vi "FPGA_XYMoving.vi"() -> ()   [LabVIEW 2014]
uses:
  <vilib>/rvi/Emulation/niFpgaSctlEmulationGetInTimedLoop.vi
  <vilib>/rvi/Emulation/niFpgaProcessEmulError.vi
  <vilib>/rvi/Memory/Memory_Emulation/nirvimemoryFastEmulation.vi
  <vilib>/rvi/Memory/Memory_Emulation/nirvimemoryEmulation.vi
  <vilib>/rvi/Emulation/niFpgaEmulationIsFPGAContextNoSignature.vi
  <vilib>/rvi/DataTransferAndStorage/Container/Common/niFpgaContainerGetUniqueNameForEmu.vi
  <vilib>/rvi/errors/nirviReportUnexpectedCaseInternalError (U32).vi
  <vilib>/rvi/eio/common/nirviEmuTemplateMethod_errors.vi
  <vilib>/rvi/Emulation/niFpgaGetClockAttributes.vi
  <vilib>/rvi/Emulation/niFpgaEmulationReportErrorSimple.vi
  <vilib>/rvi/occurrence/nirviWaitOnOccurrenceBase.vi
  <vilib>/rvi/Emulation/niFpgaCriticalErrorInLSC.vi
  <vilib>/rvi/DataTransferAndStorage/Container/XNode/niFpgaContainer.xnode
  <vilib>/eio/EIONode/EIONode.xnode
panel:
  out "DIO 0":bool
  out "XPresNum":i32
  out "YPresNum":i32
  in  "YOffset":i16
  in  "XOffset":i16
  in  "YStepIndex":i16
  in  "XStepIndex":i16
  in  "stop":bool
  in  "YNum":i16
  in  "XNum":i16
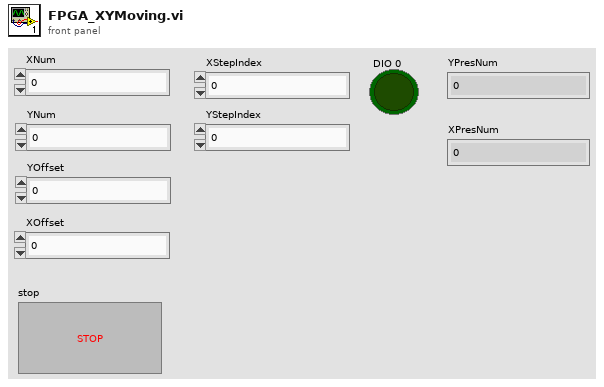
[diagram p1: front panel]
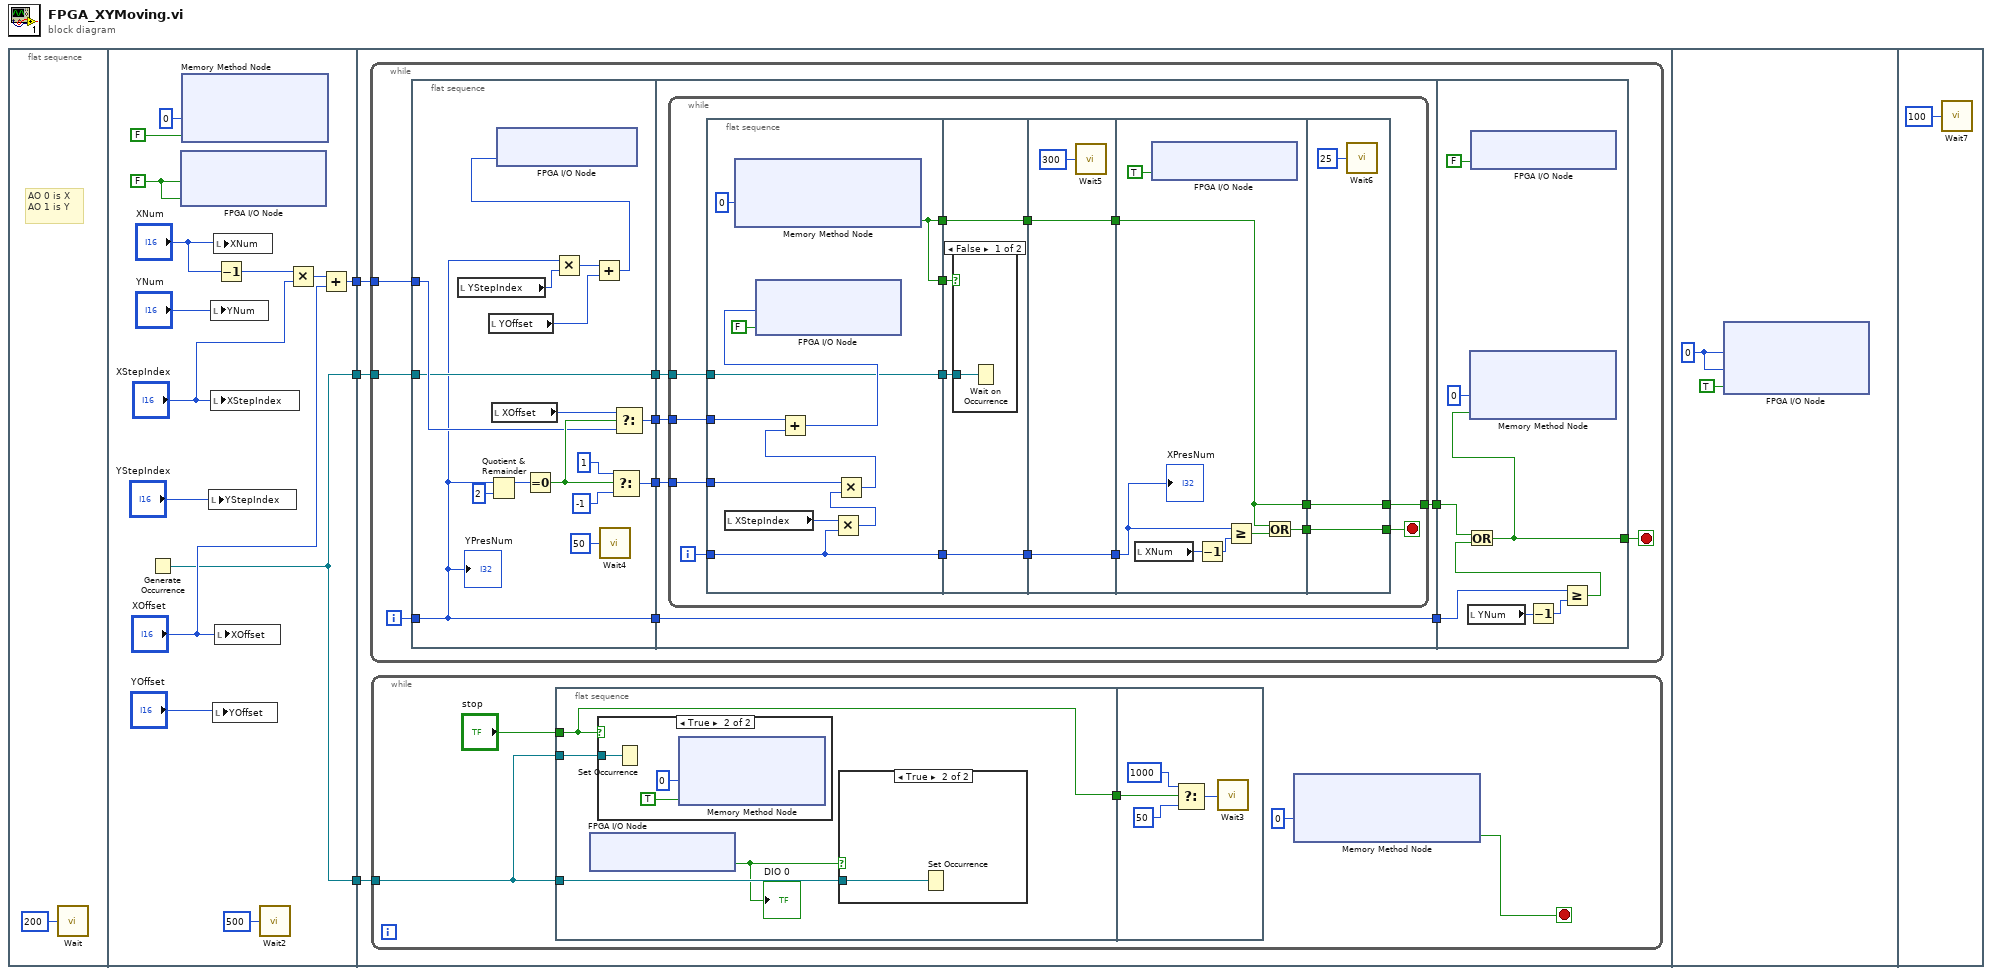
[diagram p0: block diagram]
diagram:
  n1 = flat-sequence {
    tunnel: [w6] -> w3
    tunnel: [w7] -> w2
    tunnel: [w6] -> w1
    tunnel: w3 -> [w21]
    tunnel: w2 -> [w20]
    tunnel: w1 -> [w19]
    frame #0 {
      # "AO 0 is X\nAO 1 is Y"
      n2 = call "Wait"("Count(mSec)"=u32 200) -> ()  [unwired: 1 out]
    }
    frame #1 {
      w5 = FALSE ("Connector0/DIO1")
      n3 = Generate Occurrence() -> (w6:refnum<k4>)
      n4 = xnode "FPGA I/O Node"("Connector0/DIO1"=w5, "Connector0/DIO2"=w5) -> ()  [unwired: 2 in, 2 out]
      n5 = xnode ("Memory Method Node")("Address"=u32 0, "Data"=FALSE) -> ()  [unwired: 1 in, 1 out]
      n6 = local write "YStepIndex"("YStepIndex") -> ()
      n7 = local write "YNum"("YNum") -> ()
      n8 = local write "XStepIndex"("XStepIndex") -> ()
      n9 = local write "YOffset"("YOffset") -> ()
      n10 = local write "XNum"("XNum") -> ()
      n11 = local write "XOffset"("XOffset") -> ()
      n12 = Decrement(x="XNum") -> (x-1=w10:i16)
      n13 = call "Wait2"("Count(uSec)"=u32 500) -> ()  [unwired: 1 out]
      n14 = Multiply(x=w10, y="XStepIndex") -> (x*y=w9:i16)
      n15 = Add(x=w9, y="XOffset") -> (x+y=w7:i16)
    }
    frame #2 {
      n16 = while {
        tunnel: w20 -> [w47]
        tunnel: w19 -> [w44]
        i -> [w48]
        stop <- w39 stop-if-true
        n17 = flat-sequence {
          tunnel: w48 -> [w49]
          tunnel: w47 -> [w60]
          tunnel: [w54] -> w46
          tunnel: [w51] -> w45
          tunnel: w44 -> [w50]
          tunnel: [w50] -> w43
          tunnel: [w49] -> w42
          tunnel: w46 -> [w69]
          tunnel: w45 -> [w68]
          tunnel: w43 -> [w67]
          tunnel: w42 -> [w66]
          tunnel: [w66] -> w41
          tunnel: [w65] -> w40
          tunnel: w41 -> [w122]
          tunnel: w40 -> [w118]
          tunnel: [w116] -> w39
          frame #0 {
            n18 = local read "YStepIndex"() -> (w58:i16)
            n19 = local read "YOffset"() -> (w56:i16)
            n20 = Quotient & Remainder(x=w49, y=2) -> (x-y*floor(x/y)=w62:i32)  [unwired: 1 out]
            n21 = local read "XOffset"() -> (w59:i16)
            n22 = Equal To 0?(x=w62) -> (x = 0?=w61:bool)
            n23 = Multiply(x=w49, y=w58) -> (x*y=w57:i32)
            n24 = Add(x=w57, y=w56) -> (x+y=w55:i32)
            n25 = xnode "FPGA I/O Node"("Connector0/AO1"=w55) -> ()  [unwired: 1 in, 1 out]
            n26 = call "Wait4"("Count(uSec)"=u32 50) -> ()  [unwired: 1 out]
            n27 = Select(t=1 ("y"), s=w61, f=-1 ("y")) -> (s? t:f=w51:i32)
            n28 = Select(t=w59, s=w61, f=w60) -> (s? t:f=w54:i16)
            "YPresNum" <- w49
          }
          frame #1 {
            n29 = while {
              tunnel: w69 -> [w83]
              tunnel: w68 -> [w84]
              tunnel: w67 -> [w82]
              tunnel: [w75] -> w65
              i -> [w85]
              stop <- w77 stop-if-true
              n30 = flat-sequence {
                tunnel: w85 -> [w88]
                tunnel: w84 -> [w94]
                tunnel: w83 -> [w93]
                tunnel: w82 -> [w90]
                tunnel: [w90] -> w81
                tunnel: [w88] -> w80
                tunnel: [w86] -> w73
                tunnel: [w86] -> w71
                tunnel: w81 -> [w100]
                tunnel: w80 -> [w99]
                tunnel: [w99] -> w78
                tunnel: w73 -> [w98]
                tunnel: [w97] -> w72
                tunnel: w71 -> [w97]
                tunnel: [w103] -> w79
                tunnel: w78 -> [w103]
                tunnel: w72 -> [w102]
                tunnel: [w102] -> w70
                tunnel: w79 -> [w110]
                tunnel: [w106] -> w76
                tunnel: [w105] -> w74
                tunnel: w70 -> [w105]
                tunnel: [w113] -> w77
                tunnel: w76 -> [w113]
                tunnel: [w112] -> w75
                tunnel: w74 -> [w112]
                frame #0 {
                  n31 = local read "XStepIndex"() -> (w96:i16)
                  n32 = xnode ("Memory Method Node")("Address"=u32 0) -> ("Data"=w86:bool)  [unwired: 1 in, 1 out]
                  n33 = Multiply(x=w96, y=w88) -> (x*y=w95:i32)
                  n34 = Multiply(x=w94, y=w95) -> (x*y=w92:i32)
                  n35 = Add(x=w93, y=w92) -> (x+y=w91:i32)
                  n36 = xnode "FPGA I/O Node"("Connector0/AO0"=w91, "Connector0/DIO1"=FALSE) -> ()  [unwired: 2 in, 2 out]
                }
                frame #1 {
                  n37 = case shown="False" w98 {
                    tunnel: w100 -> [w101 _]
                    frame False {
                      n38 = Wait on Occurrence(2:w101) -> ()  [unwired: 2 in, 1 out]
                    }
                    frame True {
                    }
                  }
                }
                frame #2 {
                  n39 = call "Wait5"("Count(uSec)"=u32 300) -> ()  [unwired: 1 out]
                }
                frame #3 {
                  n40 = local read "XNum"() -> (w108:i16)
                  n41 = xnode "FPGA I/O Node"("Connector0/DIO1"=TRUE) -> ()  [unwired: 1 in, 1 out]
                  n42 = Decrement(x=w108) -> (x-1=w109:i16)
                  n43 = Greater Or Equal?(x=w110, y=w109) -> (x >= y?=w107:bool)
                  n44 = Or(x=w105, y=w107) -> (x .or. y?=w106:bool)
                  "XPresNum" <- w110
                }
                frame #4 {
                  n45 = call "Wait6"("Count(uSec)"=u32 25) -> ()  [unwired: 1 out]
                }
              }
            }
          }
          frame #2 {
            n46 = local read "YNum"() -> (w119:i16)
            n47 = xnode "FPGA I/O Node"("Connector0/DIO1"=FALSE) -> ()  [unwired: 1 in, 1 out]
            n48 = Decrement(x=w119) -> (x-1=w120:i16)
            n49 = Greater Or Equal?(x=w122, y=w120) -> (x >= y?=w117:bool)
            n50 = Or(x=w118, y=w117) -> (x .or. y?=w116:bool)
            n51 = xnode ("Memory Method Node")("Address"=u32 0, "Data"=w116) -> ()  [unwired: 1 in, 1 out]
          }
        }
      }
      n52 = while {
        tunnel: w21 -> [w22]
        stop <- w24 stop-if-true
        n53 = flat-sequence {
          tunnel: "stop" -> [w28]
          tunnel: w22 -> [w30]
          tunnel: [w28] -> w23
          tunnel: w22 -> [w27]
          tunnel: w23 -> [w38]
          frame #0 {
            n54 = xnode "FPGA I/O Node"() -> ("Connector0/DIO0"=w29:bool)  [unwired: 1 in, 1 out]
            "DIO 0" <- w29
            n55 = case shown="True" w28 {
              tunnel: w27 -> [_ w32]
              frame False {
              }
              frame True {
                n56 = Set Occurrence(w32) -> ()
                n57 = xnode ("Memory Method Node")("Address"=u32 0, "Data"=TRUE) -> ()  [unwired: 1 in, 1 out]
              }
            }
            n58 = case shown="True" w29 {
              tunnel: w30 -> [_ w31]
              frame False {
              }
              frame True {
                n59 = Set Occurrence(w31) -> ()
              }
            }
          }
          frame #1 {
            n60 = Select(t=u32 1000, s=w38, f=u32 50 ("Count(uSec)")) -> (s? t:f=w36:u32)
            n61 = call "Wait3"("Count(uSec)"=w36) -> ()  [unwired: 1 out]
          }
        }
        n62 = xnode ("Memory Method Node")("Address"=u32 0) -> ("Data"=w24:bool)  [unwired: 1 in, 1 out]
      }
    }
    frame #3 {
      w124 = i16 0 ("Connector0/AO0")
      n63 = xnode "FPGA I/O Node"("Connector0/AO0"=w124, "Connector0/AO1"=w124, "Connector0/DIO2"=TRUE) -> ()  [unwired: 3 in, 3 out]
    }
    frame #4 {
      n64 = call "Wait7"("Count(uSec)"=u32 100) -> ()  [unwired: 1 out]
    }
  }
